vi "SystemToggleSuspensionControl (1).vi"(11 "SuspensionOn?":bool) -> (3 "SuspensionToggle Complete":bool)   [LabVIEW 2017]
doc: "Enables or disables Suspension in optimal order to prevent unneccessary air loss. Also ensures that, when present, pressure will remain above desired level."
uses:
  Sensors/DataStreamIndex.ctl
  DataTargetsGLOBAL.vi
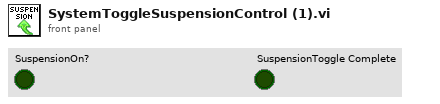
[diagram p1: front panel]
types:
  T1 = typedef "DataStreamIndex.ctl" = enum16{"SuspensionPT (PSI)", "MagBrakePT (PSI)", "Baby HPPT (PSI)", "BigRight HPPT (PSI)", "BigLeft HPPT (PSI)", "HallEffect FrontLeft (V)", "HallEffect FrontRight (V)", "HallEffect BackRight (V)", "HallEffect BackLeft (V)", "LinearPot FrontRight (V)", "LinearPot FrontLeft (V)", "LinearPot BackRight (V)", "LinearPot BackLeft (V)", "Speed (m/s)", "Distance (m)", "Piezo (V)", "Battery Voltage (V)", "Battery Current", "Battery Temperature (C)", "cRIO Temperature (C)", "Right Big Tank Temperature (C)", "Left Big Tank Temperature (C)", "Baby Tank Temperature (C)", "Right Manifold Temperature (C)", "Left Manifold Temperature (C)", "IMU Acceleration (m/s2)", "IMU Pressure (Pa)", "IMU Temperature (C)"}
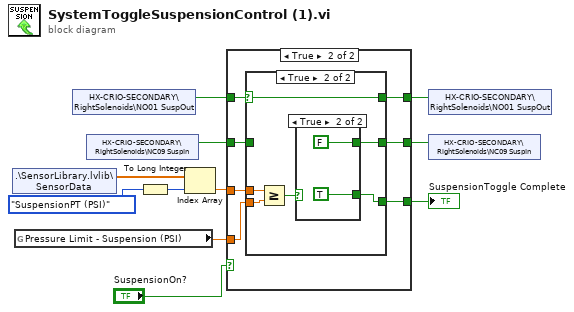
[diagram p0: block diagram]
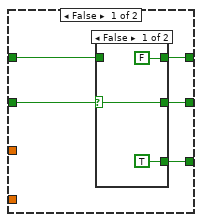
[diagram p2: hidden frame]
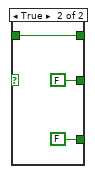
[diagram p3: hidden frame]
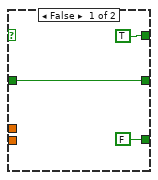
[diagram p4: hidden frame]
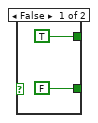
[diagram p5: hidden frame]
diagram:
  n1 = shared-variable ".\\SensorLibrary.lvlib\\SensorData"() -> (w2:dbl[])  [unwired: 1 in, 1 out]
  n2 = global read "DataTargetsGLOBAL.vi" "Pressure Limit - Suspension (PSI)"() -> (w5:dbl)
  n3 = shared-variable "HX-CRIO-SECONDARY\\RightSolenoids\\NO01 SuspOut"() -> (w7:bool)  [unwired: 1 in, 1 out]
  n4 = shared-variable "HX-CRIO-SECONDARY\\RightSolenoids\\NC09 SuspIn"() -> (w8:bool)  [unwired: 1 in, 1 out]
  n5 = To Long Integer(number=DataStreamIndex."SuspensionPT (PSI)" ("Data Stream Index")) -> (32bit integer=w4:i32)
  n6 = Index Array(array=w2, index=w4) -> (element=w1:dbl)
  n7 = case shown="True" "SuspensionOn?" {
    tunnel: w7 -> [w13 w29]
    tunnel: [w14 w28] -> w10
    tunnel: [w15 w24] -> w6
    tunnel: w8 -> [w16 w27]
    tunnel: w1 -> [_ w26]
    tunnel: [w12 w25] -> w9
    tunnel: w5 -> [_ w23]
    frame False {
      n8 = case shown="False" w16 {
        selector: w16 -> [w18 _]
        tunnel: [w18 FALSE] -> w15
        tunnel: [FALSE ("MagBrake OUTPUT") w21] -> w14
        tunnel: w13 -> [_ w21]
        tunnel: [TRUE FALSE] -> w12
        frame False {
        }
        frame True {
        }
      }
    }
    frame True {
      n9 = case shown="True" w29 {
        selector: w29 -> [_ w38]
        tunnel: [TRUE w38] -> w28
        tunnel: [w31 w37] -> w24
        tunnel: w27 -> [w31 _]
        tunnel: w26 -> [_ w36]
        tunnel: [FALSE w35] -> w25
        tunnel: w23 -> [_ w33]
        frame False {
        }
        frame True {
          n10 = Greater Or Equal?(x=w36, y=w33) -> (x >= y?=w34:bool)
          n11 = case shown="True" w34 {
            tunnel: [TRUE FALSE] -> w37
            tunnel: [FALSE TRUE] -> w35
            frame False {
            }
            frame True {
            }
          }
        }
      }
    }
  }
  "SuspensionToggle Complete" <- w9
  n12 = shared-variable "HX-CRIO-SECONDARY\\RightSolenoids\\NO01 SuspOut"(w10) -> ()  [unwired: 1 in, 1 out]
  n13 = shared-variable "HX-CRIO-SECONDARY\\RightSolenoids\\NC09 SuspIn"(w6) -> ()  [unwired: 1 in, 1 out]
